vi "Forebrain - Bill.vi"() -> ()   [LabVIEW 2012]
doc: "This VI contrains the Forebrain within the Olin Robot Architecture. It must be run first to load the appropriate mission definition files. It contains a finite state machine built around a tabbed Operator interface that will guide an operator through the startup, run shutdown mission sequence. After running it, run the Midbrain and Hindbrain VIS."
panel:
  out "NXT String Sent":string="$B^"
  in  "Soft E-Stop":bool
  out "NXT String Received":string
  out "return count":u32
  out "error out":errorcluster
  in  "error in 2":errorcluster
  out "Desired \nVelocity":i16=5
  out "Local\nHeading":i16=90
  out "Ycurrent":dbl format="%#_3g"
  out "Xcurrent":dbl format="%#_3g"
  out "Ystart":dbl
  out "Xstart":dbl
  in  "error in":errorcluster
  out "Robot Live":bool
  in  "E-Stop":bool
  in  "Tab":T1(tab)
  out "MissionTime (Min)":dbl(knob) scale=0.0..10.0
  out "LidarDist":i16
  out "IR Index":i32
  out "BatteryLevel":dbl(slide) scale=6.0..9.0
  out "String Received":string
  out "Send String":string="$B^"
  in  "VISA resource name":refnum<visa-resource-name>="COM6"
  in  "Mode":i16 min=0 max=99 step=1
  in  "Desired Vel":i16(slide)=7 scale=0.0..14.0
  in  "Local Head":i16(slide)=7 scale=0.0..14.0
  out "StartMissionMap":picture
  out "MapDARCheck":picture
  in  "RunRobot":bool
  in  "Tug letter":string="G"
  out "Tug X":i32
  out "Tug Y":i32
  out "Tug H":i32
  out "BS Time Out?":bool
  out "Buoy locations":cluster{"regular expression":string, i32, i32}[](array[cluster])
  out "Valid ?":bool
  out "Battery\nVolts":i16
  out "Base Station data rec'd":string
  out "udp rate":bool
  out "CollisionWarning":bool
  out "DebugMapDAR":picture
  in  "MapDAR Control":T2={"NumberOfBeams"=180, "SensorRange"=500.0, "Noise (0.1 to 1)"=0.0} {"Noise (0.1 to 1)" min=0.0 max=1.0 step=0.1; "SensorRange" min=500.0 max=1500.0 step=100.0; "NumberOfBeams" min=36 max=360 step=2}
  out "MapDAR Data (r:pixel b:degrees)":cluster{"Range":dbl, "Bearing":dbl}[](array[cluster])
  in  "Stop DebugSENSE":bool
  out "MissionMap":picture
  out "Tug position":T3
  out "initialized MDF":T4(array[cluster])
  out "Way Point Index":i32
  out "InitialWaypoint":cluster{"X":i16, "Y":i16}
  in  "Pen Color":u32(colorbox)=15671808
  in  "Select Pen Attributes":T5={"Width"=1, "Style"=enum."Solid"}
  out "Draw??":bool
  in  "WhereAmI?FromBase":T6
  out "(xr,yr)":cluster{"X":dbl, "Y":dbl}
  in  "RobotPosition":T3 {"xrobot" min=0.0 max=1177.0 step=10.0; "yrobot" min=0.0 max=850.0 step=10.0; "heading" min=0.0 max=7.0 step=0.1}
  out "MDF_Original":T4(array[cluster])
  out "WhatAroundMeMap?":cluster{"T":dbl, "Range":dbl, "Bearing":dbl}[](array[cluster])
  out "WayPointAct":dbl[](array[numeric])
  out "SteerAngle":dbl
  out "MissionDefFile":picture
  out "MDF":T4(array[cluster])
  in  "Select Your Behavior":T7(ring)
  out "No. of Waypoints":i32
  in  "Exit Planning":bool
  in  "BoatSpeed for Leg":dbl(slide)=8.0 min=-9.0 max=9.0 step=1.0 scale=0.0..14.0
  out "BuildMDF":bool
  out "WayPoint Position":cluster{"X":i32, "Y":i32}
  in  "Upper Midbrain Active":bool
  out "Send String to NXT":string="$B^"
  in  "Behavior Command":T7(ring)
  out "CollisionLight":bool
  out "Where? Manual":T6
  out "ActManual":bool
  in  "Manual Heading":i16(knob) min=0 max=14 step=1
  out "MWhat?":bool
  out "Where? 2":bool
  out "How? 2":bool
  in  "ManualModeStop":bool
  out "ManualModeMapDAR":picture
  out "ManualMissionMap":picture
  out "Battery":dbl(slide) scale=0.0..8.0
  in  "Manual Vel":dbl(slide) min=0.0 max=14.0 step=1.0 scale=0.0..14.0
  out "MissionTime":dbl(knob) scale=0.0..10.0
  out "Heading":cluster{dbl, dbl}(knob)={0.0, 34.390870865624734} scale=180.0..-179.0 scale format="%#_3g"
  out "Speed":i16(knob) scale=-6.0..6.0
  out "Current Behavior":T7(ring)
  out "Robot Position":cluster{"X":dbl, "Y":dbl} {"X" format="%#_3g"; "Y" format="%#_3g"}
  out "Ready":bool
  in  "Pause":bool
  in  "Rerun MDF":bool
  out "CollisionLight 2":bool
  out "Act":bool
  out "Neo-C":bool
  out "How?":bool
  out "What?":bool
  out "A Heading":cluster{dbl, dbl}(knob)={0.0, 34.390870865624734} scale=180.0..-180.0
  out "A Speed":dbl(knob) scale=-9.0..9.0
  out "AutoBattery":dbl(slide) scale=0.0..8.0
  out "AutoModeLIDAR":picture
  out "AutoMissionMap":picture
  in  "RunAutoMode":bool
  out "MissionTimeAuto":dbl(knob) scale=0.0..60.0
  out "Where?":bool
  in  "Manual Override":bool
  in  "Destinations Array":i64[][](array[numeric])
  out "BAM Mission Map":picture
  in  "Pixel Y Goal":dbl
  in  "Pixel X Goal":dbl
  out "Pixel X":dbl
  out "Pixel Y":dbl
  out "Direction":dbl
  out "Base Station String":string
  out "Battery Level":dbl
  in  "Heading":i16(knob)=7
  in  "Velocity":i16(slide)=7 scale=0.0..14.0
  # "To run\nrobot,\nclick\narrow\nabove\n\nRun Robot button must be on"
  # "Operation Directions\n\n1)Click on Startup&\nShutdown tab.\n2) Click on Run \nArrow on menubar.\nRun Forebrain,\nvis from the project\nexplorer.\n3) Select a mssion \nmap file when asked.\n4) Check robot is \nfully operational on\nStartup tab.\n5) Debug with debug\ntabs as required.\n6) Select ManualMode\ntab and test drive \nrobot.\n7) Select PlanMission\ntab and set up \nmission.\n8) Go to AutoMode\ntab and run mission."
  # "Turns off drive\nmotors"
  # "Enter Olin Test  Pool"
  # "Xbee Com Port"
  # "xBee\"Send String\" (mode, desired velocity, local heading)"
  # "(Type in Tug Letter  L T G P  (look at boat cradle)"
  # "Should be on to\nrun"
  # "BoatG,X,Y,H,BoatT,X,Y,H,BoatP,X,Y.H,BoatL,X,Y,H,BuoyA,X,Y,BuoyB,X,Y,BuoyC,X,Y,BuoyD,X,Y,Time(hours,Min,Sec)"
  # "To stop  program \nturn off here"
  # "Use this tab\nto explore\nLIDAR\ndata and \noperation"
  # "Set\nNumberOfBeams\nSensorRange\nNoise\nto\nview\nsimulated\nsensor\ndata"
  # "Turn Debug Sim \nto leave this\ntab--->"
  # "This tab will auto\nreturn to Startup \nin 2 seconds"
  # "Clean up interface and make more useful for debugging behaviors"
  # "Build out interface and make more useful for debugging act"
  # "This tab will auto\nreturn to Startup \nin 2 seconds"
  # "Directions:\n1) Select Robot Behavior for each mission leg.\n2) Select Robot Speed for leg.\n3) Click on robots current location for first waypoint.\n4) Hold down button and drag to next\nwaypoint. Click on next leg waypoint.\n5) Hold mouse button down and drag to \nnext waypoint. \n6) Click on next waypoint. Repeat for full mission.\n7) MDF will store up to 20 waypoints."
  # "Remember to\nset boat\nleg speed !"
  # "Please Adjust Scroll Barrs in Tug Off Mode to Prevent  Extra Lines Being Drawn"
  # "\"Send String\" (mode, desired velocity, local heading)"
  # "Press to stop and return to StartUp"
  # "Open MidBrain\nArbiter to see\nBrain Waves"
  # "AutoMode\nAutomatically \nReturns to \nStartUp Mode"
  # "Pixel coordinates for destinations."
  # "BoatG,X,Y,H,BoatT,X,Y,H,BoatP,X,Y.H,BoatL,X,Y,H,BuoyA,X,Y,BuoyB,X,Y,BuoyC,X,Y,BuoyD,X,Y,Time(hours,Min,Sec)"
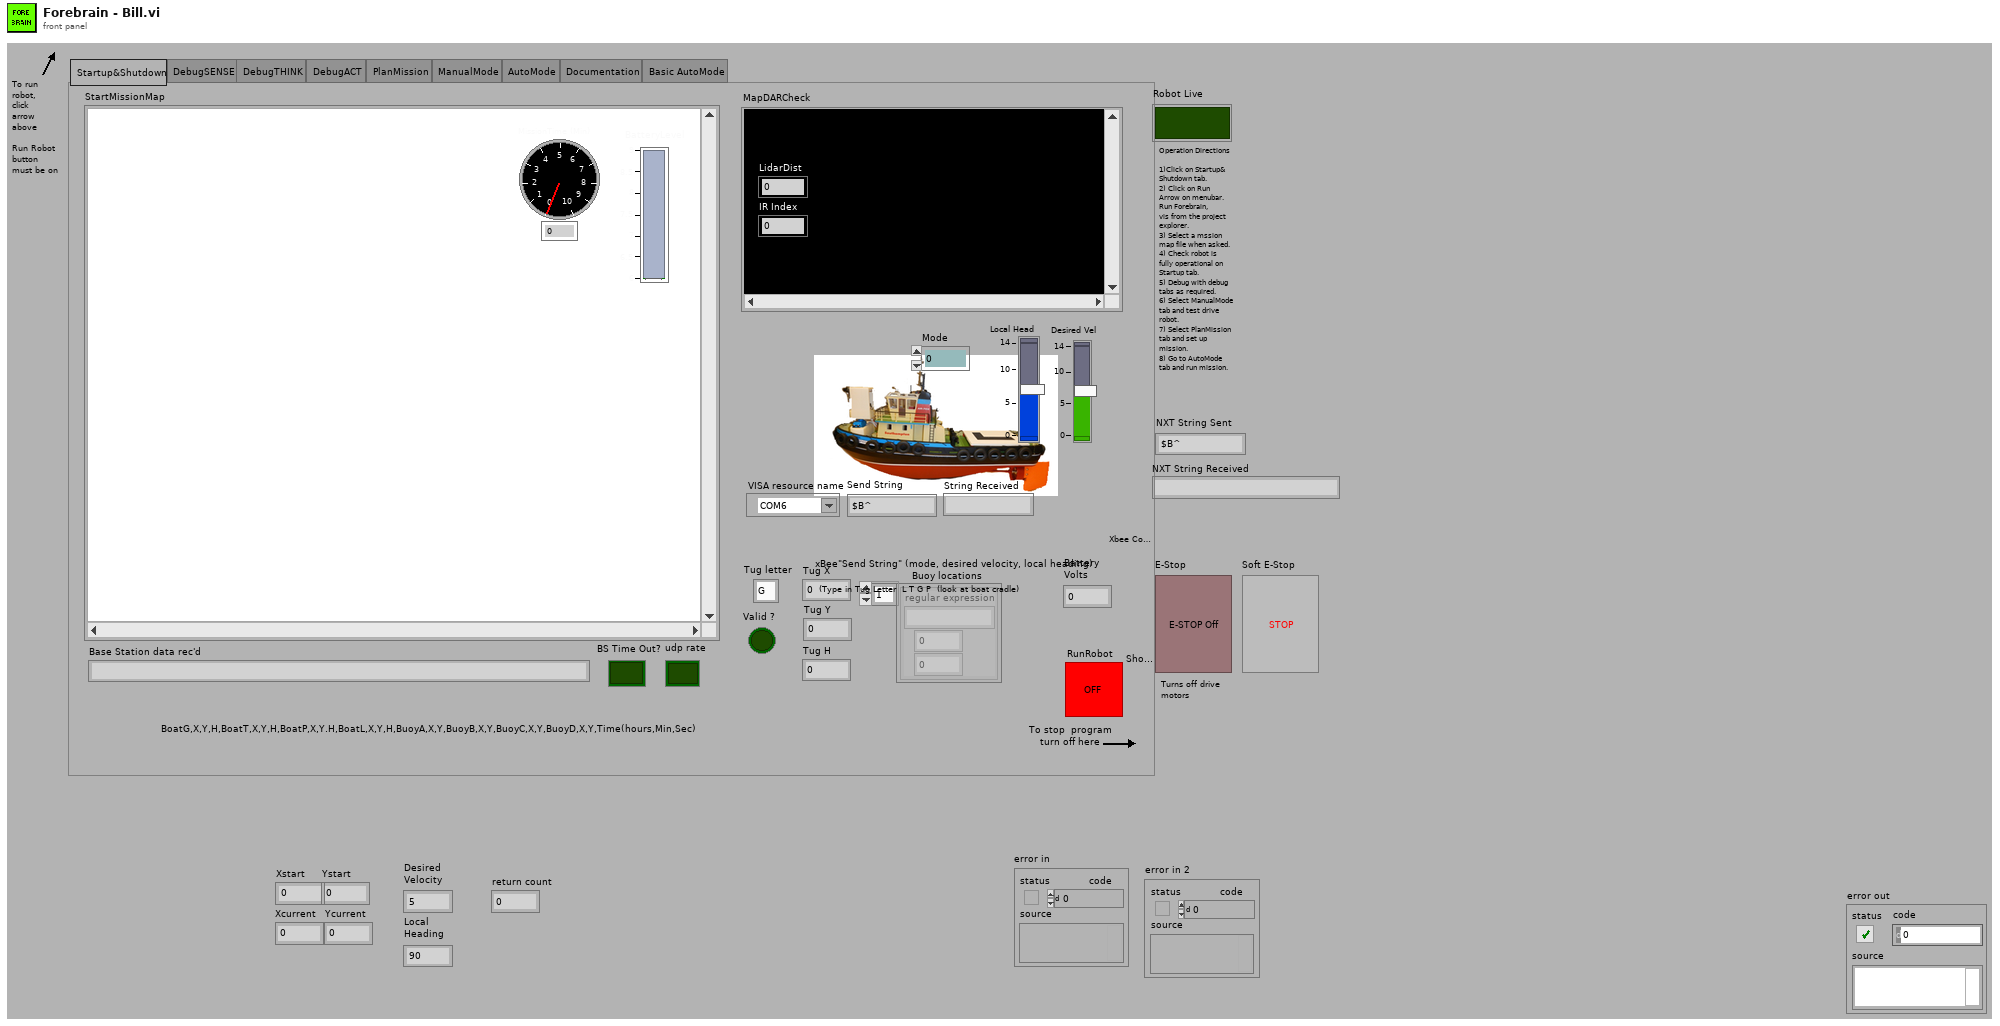
[diagram p1: front panel]
types:
  T1 = enum32{"Startup&Shutdown", "DebugSENSE", "DebugTHINK", "DebugACT", "PlanMission", "ManualMode", "AutoMode", "Documentation", "Basic AutoMode"}
  T2 = cluster{"NumberOfBeams":i32, "SensorRange":dbl, "Noise (0.1 to 1)":dbl}
  T3 = cluster{"xrobot":dbl, "yrobot":dbl, "heading":dbl}
  T4 = cluster{"Status":enum16{"Past", "Current", "Future"}, "x":dbl, "y":dbl, "z":dbl, "Vel":dbl, "Dwell Time":dbl, "BehCom":enum16{"Tug Off", "Manual Mode", "Goto WayPoint", "Back Up", "Circle", "Left Wall Follow", "Right Wall Follow", "Hunt"}, "Expand1":dbl, "Expand2":dbl, "Expand3":dbl}[]
  T5 = cluster{"Width":u16, "Style":enum32{"Solid", "Dash", "Dot", "DashDot", "DashDotDot"}}
  T6 = cluster{"T":dbl, "X":dbl, "Y":dbl, "Direction":dbl}
  T7 = enum16{"Tug Off", "Manual Mode", "Goto WayPoint", "Back Up", "Circle", "Left Wall Follow", "Right Wall Follow", "Hunt"}
  T8 = enum32{"Startup&Shutdown", "DebugSENSE", "DebugTHINK", "DebugACT", "PlanMission", "ManualMode", "AutoMode", "Documentation"}
  T9 = cluster{"VelCom":dbl, "BehCom":enum16{"OpenFieldTransit", "P-WallFollow", "S-WallFollow", "LaneFollow", "ManualMode"}}
  T10 = typedef "IMAQ Image.ctl" = refnum<image>
  T11 = typedef "imagedata.ctl" = cluster{"image type":i32, "image depth":i32, "image":u8[], "mask":u8[], "colors":u32[], "Rectangle":cluster{"left":i16, "top":i16, "right":i16, "bottom":i16}}
  T12 = cluster{"Status":enum16{"Past", "Current", "Future"}, "x":dbl, "y":dbl, "z":dbl, "Vel":dbl, "Dwell Time":dbl, "BehCom":enum16{"Tug Off", "Manual Mode", "Goto WayPoint", "Back Up", "Circle", "Left Wall Follow", "Right Wall Follow", "Hunt"}, "Expand1":dbl, "Expand2":dbl, "Expand3":dbl}
  T13 = typedef "LVMouseTypeDef.ctl" = cluster{"Mouse Position":cluster{"X":i32, "Y":i32}, "Mouse Modifiers":cluster{"Button Down":bool, "Shift Mod":bool, "Menu Mod":bool, "Option Mod":bool}}
  T14 = cluster{"regular expression":string, i32, i32, i32}
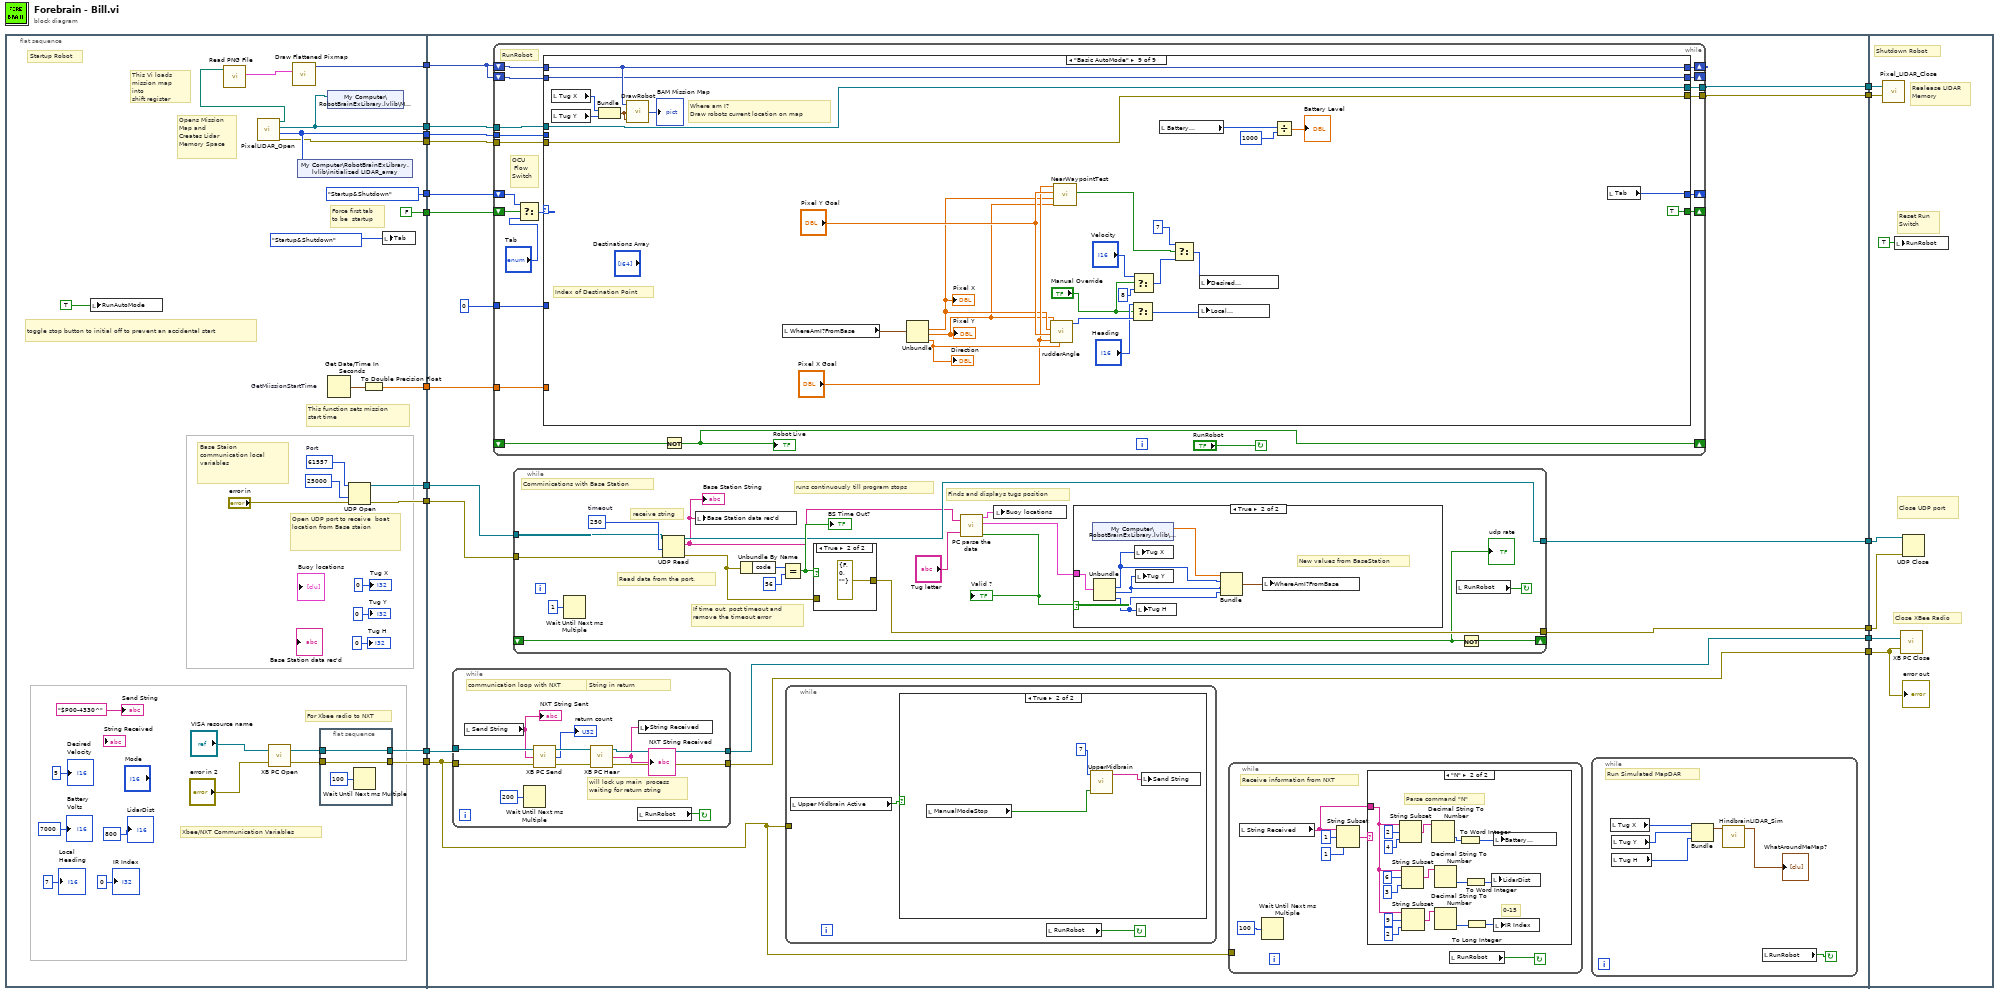
[diagram p0: block diagram]
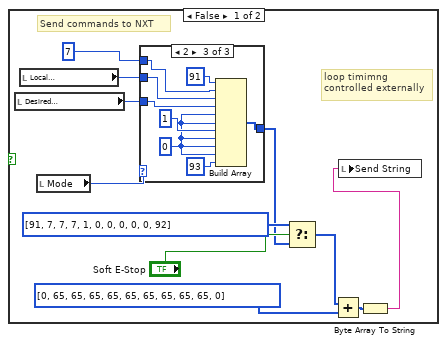
[diagram p3: hidden frame]
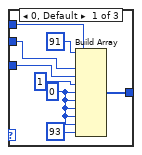
[diagram p4: hidden frame]
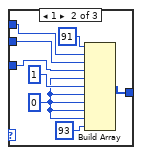
[diagram p5: hidden frame]
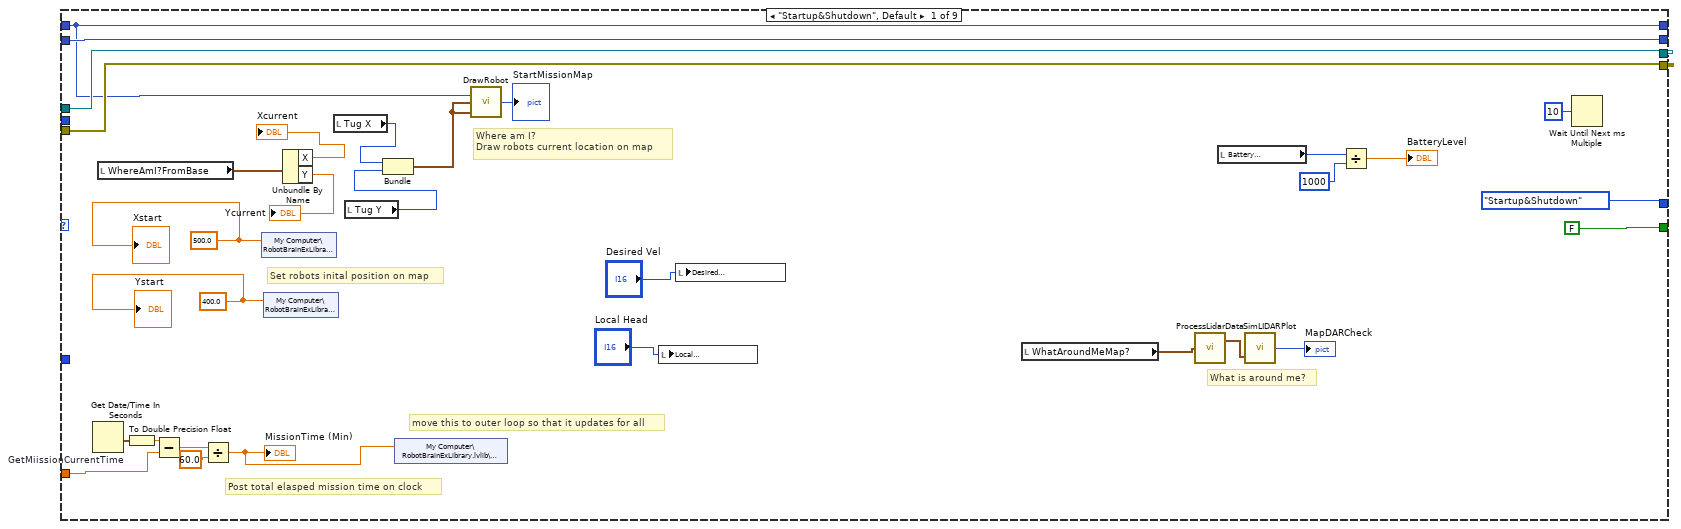
[diagram p8: hidden frame]
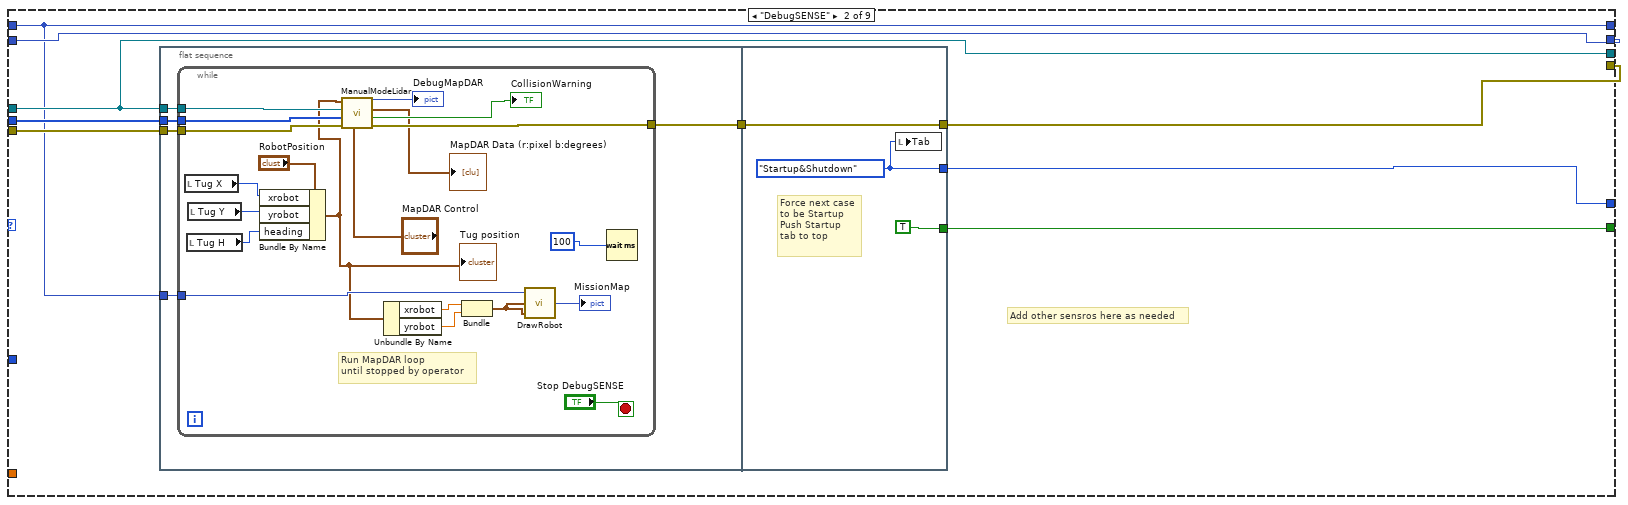
[diagram p9: hidden frame]
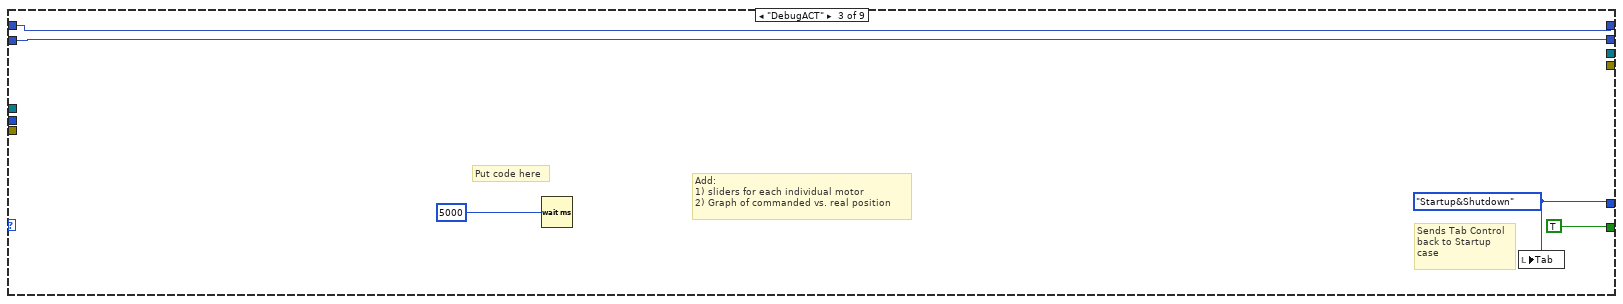
[diagram p10: hidden frame]
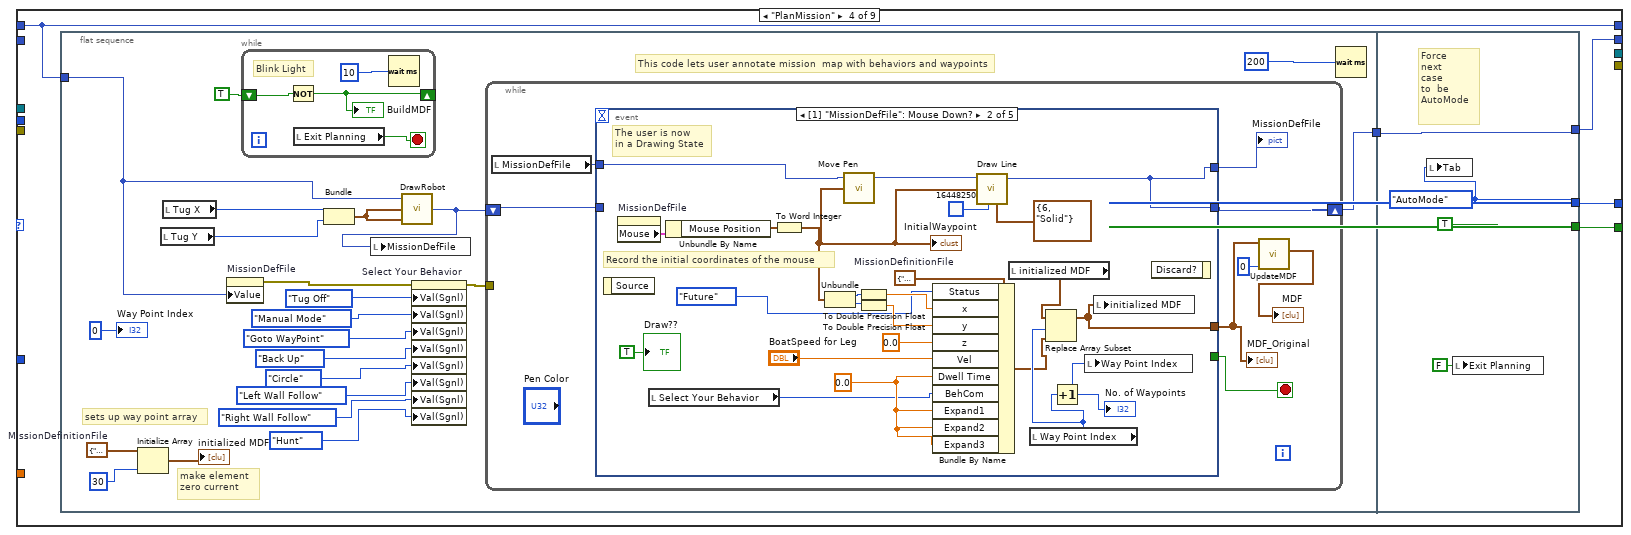
[diagram p11: hidden frame]
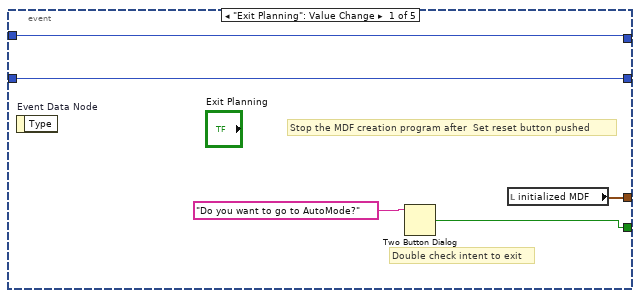
[diagram p12: hidden frame]
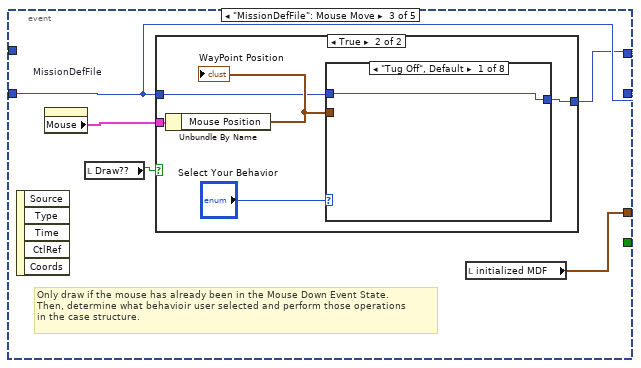
[diagram p13: hidden frame]
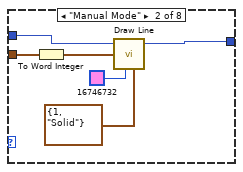
[diagram p15: hidden frame]
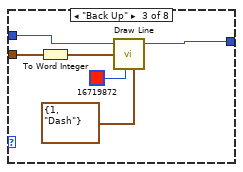
[diagram p16: hidden frame]
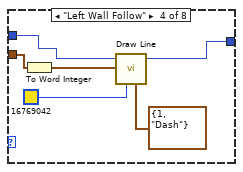
[diagram p17: hidden frame]
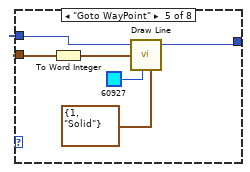
[diagram p18: hidden frame]
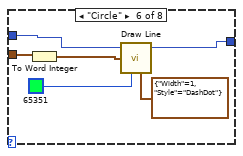
[diagram p19: hidden frame]
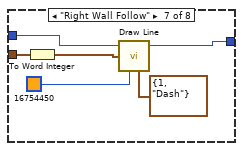
[diagram p20: hidden frame]
diagram:
  n1 = flat-sequence {
    tunnel: [w48] -> w17
    tunnel: [w47] -> w16
    tunnel: [w44] -> w15
    tunnel: [w46] -> w14
    tunnel: [w45] -> w13
    tunnel: [FALSE ("RunAutoMode")] -> w10
    tunnel: [T8."Startup&Shutdown" ("Tab")] -> w9
    tunnel: [w31] -> w8
    tunnel: [w30] -> w7
    tunnel: [w19] -> w6
    tunnel: [w18] -> w5
    tunnel: w17 -> [w70]
    tunnel: w16 -> [w69]
    tunnel: w15 -> [w68]
    tunnel: w14 -> [w67]
    tunnel: w13 -> [w66]
    tunnel: [w65] -> w12
    tunnel: [w64] -> w11
    tunnel: w10 -> [w63]
    tunnel: w9 -> [w62]
    tunnel: w8 -> [w57]
    tunnel: w7 -> [w56]
    tunnel: w6 -> [w61]
    tunnel: w5 -> [w58]
    tunnel: [w60] -> w4
    tunnel: [w59] -> w3
    tunnel: [w55] -> w2
    tunnel: [w54] -> w1
    tunnel: w12 -> [w647]
    tunnel: w11 -> [w646]
    tunnel: w4 -> [w645]
    tunnel: w3 -> [w644]
    tunnel: w2 -> [w643]
    tunnel: w1 -> [w642]
    frame #0 {
      w37 = u16 61557  # Port
      # "For Xbee radio to NXT"
      # "Xbee/NXT Communication Variables"
      # "Base Staion communication local variables"
      # "Open UDP port to receive  boat location from Base staion"
      # "Force first tab\nto be  startup"
      # "toggle stop button to initial off to prevent an accidental start"
      # "Opens Mission\nMap and\nCreates Lidar\nMemory Space"
      # "This function sets mission \nstart time"
      # "This Vi loads\nmission map into \nshift register"
      # "Startup Robot"
      n2 = local write "RunAutoMode"(TRUE ("RunAutoMode")) -> ()
      n3 = call "PixelLIDAR_Open.vi"() -> ("error out"=w45:errorcluster, "initialized LIDAR\narray"=w46:i32[], "MDF Image"=w44:T10, "MissionMap"=w39:path)  [unwired: 2 in]
      n4 = call <vilib>:"Read PNG File.vi"("path to PNG file"=w39) -> ("image data"=w38:T11)  [unwired: 8 in, 2 out]
      n5 = call "XB PC Open.vi"("error in (no error)"="error in 2", "VISA resource name"="VISA resource name") -> ("error out"=w22:errorcluster, "VISA resource name out"=w23:refnum<visa-resource-name>)
      n6 = call <vilib>:"Draw Flattened Pixmap.vi"("image data"=w38) -> ("new picture"=w47:picture)  [unwired: 8 in]
      n7 = shared-variable "My Computer\\RobotBrainExLibrary.lvlib\\initialized LIDAR_array"(w46) -> ()  [unwired: 1 in, 1 out]
      n8 = flat-sequence {
        tunnel: w23 -> [w50]
        tunnel: w22 -> [w51]
        tunnel: [w51] -> w18
        tunnel: [w50] -> w19
        frame #0 {
          n9 = Wait Until Next ms Multiple(millisecond multiple=u32 100) -> ()  [unwired: 1 out]
        }
      }
      n10 = shared-variable "My Computer\\RobotBrainExLibrary.lvlib\\MDF Image"(w44) -> ()  [unwired: 1 in, 1 out]
      n11 = Get Date/Time In Seconds "GetMiissionStartTime"() -> (seconds since 1Jan1904=w49:timestamp)
      n12 = UDP Open(8:"error in", 9:25000 ("timeout ms (25000)"), 11:w37) -> (port=w31:refnum<k16>, 0:w30:errorcluster)  [unwired: 2 in, 1 out]
      n13 = To Double Precision Float(number=w49) -> (double precision float=w48:dbl)
      n14 = local write "Tab"(T8."Startup&Shutdown" ("Tab")) -> ()
      "Tug X" <- 0 ("Tug X")
      "Tug Y" <- 0 ("Tug Y")
      "Tug H" <- 0 ("Tug H")
      "Battery\nVolts" <- i16 7000 ("Battery\nVolts")
      "LidarDist" <- i16 800 ("Dist")
      "IR Index" <- 0 ("IR Index")
      "Local\nHeading" <- i16 7 ("Local\nHeading")
      "Desired \nVelocity" <- i16 5 ("Desired \nVelocity")
      "Send String" <- "$P00-4330^"
    }
    frame #1 {
      n15 = while {
        tunnel: w61 -> [w149]
        tunnel: w58 -> [w148]
        tunnel: [w145] -> w59
        tunnel: [w144] -> w60
        stop <- w143 continue-if-true
        # "will lock up main  process\nwaiting for return string"
        # "communication loop with NXT"
        # "send a string to the NXT and receive a String in return"
        n16 = local read "Send String"() -> (w141:string)
        "NXT String Sent" <- w141
        n17 = Wait Until Next ms Multiple(millisecond multiple=u32 200) -> ()  [unwired: 1 out]
        n18 = call "XB PC Send.vi"("error in (no error)"=w148, "String"=w141, "VISA resource name"=w149) -> ("error out"=w147:errorcluster, "return count"=→"return count":u32, "VISA resource name out"=w146:refnum<visa-resource-name>)
        n19 = call "XB PC Hear.vi"("VISA resource name"=w146, "error in (no error)"=w147) -> ("VISA resource name out"=w144:refnum<visa-resource-name>, "String Received"=w140:string, "error out"=w145:errorcluster)
        "NXT String Received" <- w140
        n20 = local read "RunRobot"() -> (w143:bool)
        n21 = local write "String Received"(w140) -> ()
      }
      n22 = while {
        shift-right: [w178] -> _
        shift-left: _ -> [w194]
        shift-right: [w193] -> _
        shift-left: w62 -> [w192]
        shift-right: [w189] -> _
        shift-left: w63 -> [w188]
        tunnel: w70 -> [w187]
        shift-right: [w177] -> _
        shift-left: w69 -> [w186]
        shift-right: [w184] -> _
        shift-left: w69 -> [w185]
        tunnel: w68 -> [w183]
        tunnel: w67 -> [w182]
        tunnel: w66 -> [w181]
        tunnel: [w180] -> w65
        tunnel: [w179] -> w64
        tunnel: 0 -> [w176]
        stop <- "RunRobot" continue-if-true
        # "RunRobot"
        # "OCU\n Flow\nSwitch"
        n23 = Select(t=w192, s=w188, f="Tab") -> (s? t:f=w190:T1)
        n24 = case shown="\"Basic AutoMode\"" w190 {
          selector: w190 -> [_ _ _ _ _ w514 _ _ _]
          tunnel: [T8."Startup&Shutdown" ("Tab") w230 w265 w272 w439 w515 T8."Startup&Shutdown" ("Tab") w611 w629] -> w193
          tunnel: [FALSE ("s") w229 TRUE ("s") w271 w440 w513 FALSE ("s") TRUE ("s") TRUE ("s")] -> w189
          tunnel: w187 -> [w219 _ _ _ w437 w511 _ _ _]
          tunnel: w186 -> [w196 w226 w264 w268 w435 w508 w604 w609 w635]
          tunnel: w185 -> [w218 w227 w263 _ w436 w510 w603 w608 w634]
          tunnel: [w218 w227 w263 w269 w436 w510 w603 w608 w634] -> w184
          tunnel: w183 -> [w217 w228 _ _ _ _ _ _ w630]
          tunnel: w182 -> [_ w234 _ _ _ _ _ _ _]
          tunnel: w181 -> [w216 w233 _ _ _ _ _ _ w627]
          tunnel: [w217 w228 _ _ _ _ _ _ w630] -> w180
          tunnel: [w216 w232 _ _ _ _ _ _ w627] -> w179
          tunnel: [w196 w226 w264 w268 w435 w508 w604 w609 w635] -> w177
          tunnel: w176 -> [_ _ _ _ _ _ _ _ _]
          frame "Startup&Shutdown", Default {
            w208 = 400.0 ("Ystart")
            w209 = 500.0 ("Xstart")
            # "move this to outer loop so that it updates for all"
            # "Where am I?\nDraw robots current location on map"
            # "Post total elasped mission time on clock"
            # "What is around me?"
            # "Set robots inital position on map"
            n25 = Get Date/Time In Seconds "GetMiissionCurrentTime"() -> (seconds since 1Jan1904=w223:timestamp)
            n26 = local read "WhereAmI?FromBase"() -> (w197:T6)
            n27 = To Double Precision Float(number=w223) -> (double precision float=w222:dbl)
            n28 = Subtract(x=w222, y=w219) -> (x-y=w221:dbl)
            n29 = Divide(x=w221, y=60.0) -> (x/y=w215:dbl)
            "MissionTime (Min)" <- w215
            n30 = shared-variable "My Computer\\RobotBrainExLibrary.lvlib\\Xstart"(w209) -> ()  [unwired: 1 in, 1 out]
            n31 = shared-variable "My Computer\\RobotBrainExLibrary.lvlib\\Ystart"(w208) -> ()  [unwired: 1 in, 1 out]
            n32 = Unbundle By Name(w197) -> ("X"=→"Xcurrent":dbl, "Y"=→"Ycurrent":dbl)
            n33 = local read "Tug X"() -> (w207:i32)
            n34 = local read "Tug Y"() -> (w206:i32)
            n35 = Bundle("Tug X"=w207, "Tug Y"=w206) -> (w212:cluster{"Tug X":i32, "Tug Y":i32})  [unwired: 1 in]
            n36 = shared-variable "My Computer\\RobotBrainExLibrary.lvlib\\MissionTime"(w215) -> ()  [unwired: 1 in, 1 out]
            n37 = call "DrawRobot.vi"("(xr,yr) old"=w212, "(xr,yr) new"=w212, "2D Picture"=w196) -> ("new picture"=→"StartMissionMap":picture)
            n38 = local write "Local\nHeading"("Local Head") -> ()
            n39 = local write "Desired \nVelocity"("Desired Vel") -> ()
            n40 = local read "WhatAroundMeMap?"() -> (w198:cluster{"T":dbl, "Range":dbl, "Bearing":dbl}[])
            n41 = call "ProcessLidarData.vi"("WhatAroundMe?MM"=w198) -> ("data array [mag, phase (deg)]"=w213:cluster{"magnitude":dbl, "phase":dbl}[])  [unwired: 1 out]
            n42 = local read "Battery\nVolts"() -> (w203:i16)
            n43 = call "SimLIDARPlot.vi"("data array [mag, phase (deg)]"=w213) -> ("SONAR"=→"MapDARCheck":picture)  [unwired: 1 in]
            n44 = Divide(x=w203, y=i16 1000) -> (x/y=→"BatteryLevel":dbl)
            n45 = Wait Until Next ms Multiple(millisecond multiple=u32 10) -> ()  [unwired: 1 out]
            "Xstart" <- w209
            "Ystart" <- w208
          }
          frame "DebugSENSE" {
            # "Add other sensros here as needed"
            n46 = flat-sequence {
              tunnel: w234 -> [w239]
              tunnel: w233 -> [w238]
              tunnel: w228 -> [w237]
              tunnel: [w236] -> w231
              tunnel: w226 -> [w235]
              tunnel: [w262] -> w232
              tunnel: w231 -> [w262]
              tunnel: [w261] -> w230
              tunnel: [TRUE ("s")] -> w229
              frame #0 {
                n47 = while {
                  tunnel: w239 -> [w259]
                  tunnel: w238 -> [w258]
                  tunnel: w237 -> [w257]
                  tunnel: [w256] -> w236
                  tunnel: w235 -> [w250]
                  stop <- "Stop DebugSENSE" stop-if-true
                  # "Run MapDAR loop\nuntil stopped by operator"
                  n48 = local read "Tug X"() -> (w244:i32)
                  n49 = local read "Tug H"() -> (w245:i32)
                  n50 = local read "Tug Y"() -> (w243:i32)
                  n51 = Bundle By Name(cluster="RobotPosition", "xrobot"=w244, "yrobot"=w243, "heading"=w245) -> (w241:T3)
                  "Tug position" <- w241
                  n52 = call "ManualModeLidar.vi"("LIDARControl"="MapDAR Control", "error in"=w258, "initialized \nsonar ray\narray"=w259, "MDF Image"=w257, "SubPosition"=w241) -> ("error out"=w256:errorcluster, "Collision\nWarning"=→"CollisionWarning":bool, "LIDAR Data (r:pixel b:degrees)"=→"MapDAR Data (r:pixel b:degrees)":cluster{"Range":dbl, "Bearing":dbl}[], "LIDAR"=→"DebugMapDAR":picture)  [unwired: 1 in]
                  n53 = Unbundle By Name(w241) -> ("xrobot"=w248:dbl, "yrobot"=w247:dbl)
                  n54 = Bundle("xrobot"=w248, "yrobot"=w247) -> (w240:cluster{"xrobot":dbl, "yrobot":dbl})  [unwired: 1 in]
                  n55 = call "DrawRobot.vi"("(xr,yr) old"=w240, "(xr,yr) new"=w240, "2D Picture"=w250) -> ("new picture"=→"MissionMap":picture)
                  n56 = Wait (ms)(milliseconds to wait=u32 100) -> ()  [unwired: 1 out]
                }
              }
              frame #1 {
                w261 = T8."Startup&Shutdown" ("Tab")
                # "Force next case\nto be Startup\nPush Startup\ntab to top"
                n57 = local write "Tab"(w261) -> ()
              }
            }
          }
          frame "DebugACT" {
            w265 = T8."Startup&Shutdown" ("Tab")
            # "Add:\n1) sliders for each individual motor\n2) Graph of commanded vs. real position"
            # "Put code here"
            # "Sends Tab Control\nback to Startup\ncase"
            n58 = Wait (ms)(milliseconds to wait=u32 5000) -> ()  [unwired: 1 out]
            n59 = local write "Tab"(w265) -> ()
          }
          frame "PlanMission" {
            n60 = flat-sequence {
              tunnel: [w293] -> w270
              tunnel: w268 -> [w286]
              tunnel: [w433] -> w272
              tunnel: [TRUE ("s")] -> w271
              tunnel: w270 -> [w432]
              tunnel: [w432] -> w269
              frame #0 {
                w284 = T12 {"Status"=enum."Future", "x"=0.0, "y"=0.0, "z"=0.0, "Vel"=0.0, "Dwell Time"=0.0, "BehCom"=enum."Tug Off", "Expand1"=0.0, "Expand2"=0.0, "Expand3"=0.0}  # MissionDefinitionFile
                # "make element \nzero current"
                # "sets up way point array"
                # "This code lets user annotate mission  map with behaviors and waypoints"
                n61 = Initialize Array ("Initialize WaypointArray")(w284, 30 ("dimension size")) -> (→"initialized MDF":T4)
                n62 = local read "Tug Y"() -> (w281:i32)
                n63 = local read "Tug X"() -> (w282:i32)
                n64 = property on="MissionDefFile" class="Pict"("Value"=w286) -> (error out=w291:errorcluster)  [unwired: 2 in, 1 out]
                n65 = while {
                  shift-right: [w297] -> _
                  shift-left: TRUE -> [w298]
                  stop <- w296 stop-if-true
                  # "Blink Light"
                  n66 = Not(x=w298) -> (.not. x?=w297:bool)
                  "BuildMDF" <- w297
                  n67 = local read "Exit Planning"() -> (w296:bool)
                  n68 = Wait (ms)(milliseconds to wait=u32 10) -> ()  [unwired: 1 out]
                }
                n69 = Bundle("Tug X"=w282, "Tug Y"=w281) -> (w287:cluster{"Tug X":i32, "Tug Y":i32})  [unwired: 1 in]
                n70 = call "DrawRobot.vi"("(xr,yr) old"=w287, "(xr,yr) new"=w287, "2D Picture"=w286) -> ("new picture"=w285:picture)
                n71 = local write "MissionDefFile"(w285) -> ()
                n72 = property on="Select Your Behavior" class="Enum (strict)"(error in=w291, "Val(Sgnl)"=T7."Tug Off" ("Value (Signaling)"), "Val(Sgnl)"=T7."Manual Mode" ("Value (Signaling)"), "Val(Sgnl)"=T7."Goto WayPoint" ("Value (Signaling)"), "Val(Sgnl)"=T7."Back Up" ("Value (Signaling)"), "Val(Sgnl)"=T7."Circle" ("Value (Signaling)"), "Val(Sgnl)"=T7."Left Wall Follow" ("Value (Signaling)"), "Val(Sgnl)"=T7."Right Wall Follow" ("Value (Signaling)"), "Val(Sgnl)"=T7."Hunt" ("Value (Signaling)")) -> (error out=w292:errorcluster)  [unwired: 1 in, 1 out]
                n73 = while {
                  shift-right: [w305] -> w293
                  shift-left: w285 -> [w306]
                  tunnel: w292 -> [_]
                  stop <- w304 stop-if-true
                  n74 = local read "MissionDefFile"() -> (w303:picture)
                  n75 = event shown="[1] \"MissionDefFile\": Mouse Down?" {
                    selector: _ -> [_ _ _ _ _]
                    dyn-events: _ -> [_ _ _ _ _]
                    timeout: _ -> [_ _ _ _ _]
                    tunnel: [w309 w317 w337 w390 w428] -> w305
                    tunnel: w306 -> [w309 _ w337 w390 _]
                    tunnel: [w310 _ _ _ _] -> w304
                    tunnel: [w308 w332 w338 w392 w429] -> w300
                    tunnel: w303 -> [w307 w318 _ w391 w428]
                    tunnel: [w307 w317 w336 w391 w428] -> w302
                    event "Exit Planning": Value Change {
                      # "Double check intent to exit"
                      # "Stop the MDF creation program after  Set reset button pushed"
                      n76 = event-data "Event Data Node"() -> ()  [unwired: 1 in, 1 out]
                      n77 = Two Button Dialog(message="Do you want to go to AutoMode?") -> (T button?=w310:bool)  [unwired: 2 in]
                      n78 = local read "initialized MDF"() -> (w308:T4)
                    }
                    event "MissionDefFile": Mouse Down? {
                      w316 = T12 {"Status"=enum."Future", "x"=0.0, "y"=0.0, "z"=0.0, "Vel"=0.0, "Dwell Time"=0.0, "BehCom"=enum."Tug Off", "Expand1"=0.0, "Expand2"=0.0, "Expand3"=0.0}  # MissionDefinitionFile
                      w326 = 0.0 ("Dwell Time")
                      # "Record the initial coordinates of the mouse"
                      # "The user is now\nin a Drawing State"
                      n79 = event-data() -> ()  [unwired: 1 in, 1 out]
                      n80 = property on="MissionDefFile" class="Pict"() -> ("Mouse"=w335:T13)  [unwired: 2 in, 2 out]
                      n81 = local read "Select Your Behavior"() -> (w313:T7)
                      n82 = Unbundle By Name(w335) -> ("Mouse Position"=w333:cluster{"X":i32, "Y":i32})
                      n83 = To Word Integer(number=w333) -> (16bit integer=w321:cluster{"X":i16, "Y":i16})
                      "InitialWaypoint" <- w321
                      n84 = Unbundle(w321) -> ("X"=w330:i16, "Y"=w329:i16)
                      n85 = call <vilib>:"Move Pen.vi"("new position"=w321, "picture"=w318) -> ("new picture"=w322:picture)  [unwired: 3 in]
                      n86 = To Double Precision Float(number=w330) -> (double precision float=w328:dbl)
                      n87 = To Double Precision Float(number=w329) -> (double precision float=w327:dbl)
                      n88 = Bundle By Name(cluster=w316, "Status"=enum16{"Past", "Current", "Future"}."Future", "x"=w328, "y"=w327, "z"=0.0, "Vel"="BoatSpeed for Leg", "Dwell Time"=w326, "BehCom"=w313, "Expand1"=w326, "Expand2"=w326, "Expand3"=w326) -> (w312:T12)
                      n89 = call <vilib>:"Draw Line.vi"("picture"=w322, "end point"=w321, "color(black)"=u32 16448250, "pen"=T5 {"Width"=6, "Style"=enum."Solid"}) -> ("new picture"=w317:picture)  [unwired: 5 in]
                      n90 = local read "initialized MDF"() -> (w331:T4)
                      n91 = local read "Way Point Index"() -> (w314:i32)
                      n92 = Replace Array Subset(array=w331, new element=w312, index=w314) -> (w332:T4)
                      n93 = Increment(x=w314) -> (x+1=w334:i32)
                      "No. of Waypoints" <- w334
                      n94 = local write "Way Point Index"(w334) -> ()
                      n95 = local write "initialized MDF"(w332) -> ()
                      n96 = event-data() -> ()  [unwired: 2 in, 1 out]
                      "Draw??" <- TRUE ("Draw??")
                    }
                    event "MissionDefFile": Mouse Move {
                      # "Only draw if the mouse has already been in the Mouse Down Event State.\nThen, determine what behavioir user selected and perform those operations\nin the case structure."
                      n97 = event-data() -> ()  [unwired: 1 in, 5 out]
                      n98 = property on="MissionDefFile" class="Pict"() -> ("Mouse"=w340:T13)  [unwired: 2 in, 2 out]
                      n99 = local read "Draw??"() -> (w339:bool)
                      n100 = case shown="True" w339 {
                        tunnel: w340 -> [_ w346]
                        tunnel: w337 -> [w341 w342]
                        tunnel: [w341 w343] -> w336
                        frame False {
                        }
                        frame True {
                          n101 = Unbundle By Name(w346) -> ("Mouse Position"=w344:cluster{"X":i32, "Y":i32})
                          "WayPoint Position" <- w344
                          n102 = case shown="\"Tug Off\", Default" "Select Your Behavior" {
                            tunnel: w344 -> [_ w352 w358 w361 w367 w372 w378 w384]
                            tunnel: [w347 w353 w359 w363 w366 w373 w379 w385] -> w343
                            tunnel: w342 -> [w347 w351 w355 w364 w368 w374 w380 w386]
                            frame "Tug Off", Default {
                            }
                            frame "Manual Mode" {
                              n103 = To Word Integer(number=w352) -> (16bit integer=w348:cluster{"X":i16, "Y":i16})
                              n104 = call <vilib>:"Draw Line.vi"("picture"=w351, "end point"=w348, "color(black)"=u32 16746732, "pen"=T5 {"Width"=1, "Style"=enum."Solid"}) -> ("new picture"=w353:picture)  [unwired: 5 in]
                            }
                            frame "Back Up" {
                              n105 = To Word Integer(number=w358) -> (16bit integer=w354:cluster{"X":i16, "Y":i16})
                              n106 = call <vilib>:"Draw Line.vi"("picture"=w355, "end point"=w354, "color(black)"=u32 16719872, "pen"=T5 {"Width"=1, "Style"=enum."Dash"}) -> ("new picture"=w359:picture)  [unwired: 5 in]
                            }
                            frame "Left Wall Follow" {
                              n107 = To Word Integer(number=w361) -> (16bit integer=w362:cluster{"X":i16, "Y":i16})
                              n108 = call <vilib>:"Draw Line.vi"("picture"=w364, "end point"=w362, "color(black)"=u32 16769042, "pen"=T5 {"Width"=1, "Style"=enum."Dash"}) -> ("new picture"=w363:picture)  [unwired: 5 in]
                            }
                            frame "Goto WayPoint" {
                              n109 = To Word Integer(number=w367) -> (16bit integer=w369:cluster{"X":i16, "Y":i16})
                              n110 = call <vilib>:"Draw Line.vi"("picture"=w368, "end point"=w369, "color(black)"=u32 60927, "pen"=T5 {"Width"=1, "Style"=enum."Solid"}) -> ("new picture"=w366:picture)  [unwired: 5 in]
                            }
                            frame "Circle" {
                              n111 = To Word Integer(number=w372) -> (16bit integer=w377:cluster{"X":i16, "Y":i16})
                              n112 = call <vilib>:"Draw Line.vi"("picture"=w374, "end point"=w377, "color(black)"=u32 65351, "pen"=T5 {"Width"=1, "Style"=enum."DashDot"}) -> ("new picture"=w373:picture)  [unwired: 5 in]
                            }
                            frame "Right Wall Follow" {
                              n113 = To Word Integer(number=w378) -> (16bit integer=w383:cluster{"X":i16, "Y":i16})
                              n114 = call <vilib>:"Draw Line.vi"("picture"=w380, "end point"=w383, "color(black)"=u32 16754450, "pen"=T5 {"Width"=1, "Style"=enum."Dash"}) -> ("new picture"=w379:picture)  [unwired: 5 in]
                            }
                            frame "Hunt" {
                              n115 = To Word Integer(number=w384) -> (16bit integer=w387:cluster{"X":i16, "Y":i16})
                              n116 = call <vilib>:"Draw Line.vi"("picture"=w386, "end point"=w387, "color(black)"=u32 16720896, "pen"=T5 {"Width"=1, "Style"=enum."DashDotDot"}) -> ("new picture"=w385:picture)  [unwired: 5 in]
                            }
                          }
                        }
                      }
                      n117 = local read "initialized MDF"() -> (w338:T4)
                    }
                    event "Select Your Behavior": Value Change {
                      # "When the user selects a new operation, we disable certain controls that aren't relevant to\nthe operation that the user is performing."
                      n118 = event-data() -> ("NewVal"=w395:T7)  [unwired: 1 in]
                      n119 = property on="Select Pen Attributes" class="Clust (strict)"() -> ("Controls[]"=w394:refnum<vi>[])  [unwired: 2 in, 2 out]
                      n120 = case shown="\"Manual Mode\"" w395 {
                        tunnel: w394 -> [w399 w400 w404 w408 w412 w416 w420 w424]
                        tunnel: "Select Pen Attributes" -> [_ _ _ _ _ _ _ _]
                        frame "Manual Mode" {
                          # "All attributes are valid for this\noperation."
                          n121 = Index Array "Index Array"(array=w399, index=1) -> (element=w397:refnum<vi>)
                          n122 = property on="Property Node" class="Ctl"(reference=w397, "Disabled"=u8 0) -> ()  [unwired: 1 in, 2 out]
                        }
                        frame "Back Up" {
                          # "All attributes are valid for this\noperation."
                          n123 = Index Array(array=w400, index=1) -> (element=w402:refnum<vi>)
                          n124 = property class="Ctl"(reference=w402, "Disabled"=u8 0) -> ()  [unwired: 1 in, 2 out]
                        }
                        frame "Tug Off" {
                          # "All attributes are valid for this\noperation."
                          n125 = Index Array "Index Array"(array=w404, index=1) -> (element=w406:refnum<vi>)
                          n126 = property on="Property Node" class="Ctl"(reference=w406, "Disabled"=u8 0) -> ()  [unwired: 1 in, 2 out]
                        }
                        frame "Left Wall Follow" {
                          # "All attributes are valid for this\noperation."
                          n127 = Index Array "Index Array"(array=w408, index=1) -> (element=w410:refnum<vi>)
                          n128 = property on="Property Node" class="Ctl"(reference=w410, "Disabled"=u8 0) -> ()  [unwired: 1 in, 2 out]
                        }
                        frame "Goto WayPoint" {
                          # "All attributes are valid for this\noperation."
                          n129 = Index Array "Index Array"(array=w412, index=1) -> (element=w414:refnum<vi>)
                          n130 = property on="Property Node" class="Ctl"(reference=w414, "Disabled"=u8 0) -> ()  [unwired: 1 in, 2 out]
                        }
                        frame "Circle" {
                          # "All attributes are valid for this\noperation."
                          n131 = Index Array "Index Array"(array=w416, index=1) -> (element=w418:refnum<vi>)
                          n132 = property on="Property Node" class="Ctl"(reference=w418, "Disabled"=u8 0) -> ()  [unwired: 1 in, 2 out]
                        }
                        frame "Right Wall Follow" {
                          # "All attributes are valid for this\noperation."
                          n133 = Index Array "Index Array"(array=w420, index=1) -> (element=w422:refnum<vi>)
                          n134 = property on="Property Node" class="Ctl"(reference=w422, "Disabled"=u8 0) -> ()  [unwired: 1 in, 2 out]
                        }
                        frame "Hunt" {
                          # "All attributes are valid for this\noperation."
                          n135 = Index Array "Index Array"(array=w424, index=1) -> (element=w426:refnum<vi>)
                          n136 = property on="Property Node" class="Ctl"(reference=w426, "Disabled"=u8 0) -> ()  [unwired: 1 in, 2 out]
                        }
                      }
                      n137 = local read "initialized MDF"() -> (w392:T4)
                    }
                    event "MissionDefFile": Mouse Up {
                      # "When the user is finished drawing, we complete the operation."
                      # "Finished Drawing"
                      n138 = event-data() -> ()  [unwired: 1 in, 3 out]
                      n139 = local write "Draw??"(FALSE ("Draw??")) -> ()
                      n140 = local read "initialized MDF"() -> (w429:T4)
                    }
                  }
                  "MissionDefFile" <- w302
                  "MDF_Original" <- w300
                  n141 = call "UpdateMDF.vi"("Index"=0, "MDF_In"=w300) -> ("MDF_Out"=→"MDF":T4)  [unwired: 9 in]
                }
                n142 = Wait (ms)(milliseconds to wait=u32 200) -> ()  [unwired: 1 out]
                "Way Point Index" <- 0 ("Boundary Point Index")
              }
              frame #1 {
                w433 = T8."AutoMode" ("Tab")
                # "Force \nnext \ncase\nto  be\nAutoMode"
                n143 = local write "Tab"(w433) -> ()
                n144 = local write "Exit Planning"(FALSE ("Exit Planning")) -> ()
              }
            }
          }
          frame "ManualMode" {
            # "Removing map shift register\nfixed memory leak?"
            # "Manual Steering by dashboard heading steering wheel\nand by speed slider"
            # "This mode lets \noperator directly\ndrive robot via\nthe ManualMode\ntabbed interface"
            n145 = while {
              shift-right: [w463] -> _
              shift-left: _ -> [w462]
              tunnel: w437 -> [w455]
              shift-right: [w452] -> _
              shift-left: _ -> [w451]
              tunnel: w435 -> [w449]
              stop <- w461 stop-if-true
              # "WhereAmI?"
              n146 = Get Date/Time In Seconds "GetMiissionCurrentTime"() -> (seconds since 1Jan1904=w456:timestamp)
              n147 = call "WhereForebrainPerception.vi"("Where? Midbrain"="WhereAmI?FromBase") -> ("Where? Forebrain"=→"Where? Manual":T6, "(xr,yr)"=w452:cluster{"X":dbl, "Y":dbl}, "Direction"=w441:dbl)  [unwired: 3 in, 1 out]
              "(xr,yr)" <- w452
              n148 = local read "ManualModeStop"() -> (w461:bool)
              n149 = To Double Precision Float(number=w456) -> (double precision float=w457:dbl)
              n150 = Greater Or Equal?(x=w441, y=181.0) -> (x >= y?=w446:bool)
              n151 = local read "Manual Heading"() -> (w453:i16)
              n152 = Subtract(x=w457, y=w455) -> (x-y=w458:dbl)
              n153 = Not(x=w462) -> (.not. x?=w463:bool)
              n154 = call "DrawRobot.vi"("(xr,yr) old"=w451, "(xr,yr) new"=w452, "2D Picture"=w449) -> ("new picture"=→"ManualMissionMap":picture)
              n155 = Divide(x=w458, y=60.0) -> (x/y=w460:dbl)
              "MissionTime" <- w460
              n156 = Subtract(x=w441, y=360.0) -> (x-y=w444:dbl)
              n157 = shared-variable "My Computer\\RobotBrainExLibrary.lvlib\\MissionTime"(w460) -> ()  [unwired: 1 in, 1 out]
              n158 = Select(t=w444, s=w446, f=w441) -> (s? t:f=w443:dbl)
              n159 = Bundle("Direction"=w443, "Manual Heading"=w453) -> (→"Heading":cluster{"Direction":dbl, "Manual Heading":i16})  [unwired: 1 in]
              n160 = Wait Until Next ms Multiple(millisecond multiple=u32 100 ("milliseconds to wait")) -> ()  [unwired: 1 out]
              "Where? 2" <- w462
            }
            n161 = while {
              shift-right: [w470] -> _
              shift-left: _ -> [w471]
              stop <- "ManualModeStop" stop-if-true
              # "WhatIsAroundMe?"
              n162 = local read "WhatAroundMeMap?"() -> (w465:cluster{"T":dbl, "Range":dbl, "Bearing":dbl}[])
              n163 = call "ProcessLidarData.vi"("WhatAroundMe?MM"=w465) -> ("Collision"=w466:bool, "data array [mag, phase (deg)]"=w467:cluster{"magnitude":dbl, "phase":dbl}[])
              "CollisionLight" <- w466
              n164 = Not(x=w471) -> (.not. x?=w470:bool)
              "MWhat?" <- w470
              n165 = call "SimLIDARPlot.vi"("data array [mag, phase (deg)]"=w467) -> ("SONAR"=→"ManualModeMapDAR":picture)  [unwired: 1 in]
              n166 = case shown="True" w466 {
                frame False {
                  # "No \nBeep"
                }
                frame True {
                  n167 = call <vilib>:"Beep.vi"("use system alert? (T)"=TRUE, "duration (msec)"=u32 1000, "frequency (Hz)"=u32 900) -> ()  [unwired: 9 in]
                }
              }
              n168 = Wait Until Next ms Multiple(millisecond multiple=u32 100 ("milliseconds to wait")) -> ()  [unwired: 1 out]
            }
            n169 = while {
              shift-right: [w495] -> _
              shift-left: _ -> [w494]
              stop <- w493 stop-if-true
              # "HowAmI?"
              n170 = local read "Battery\nVolts"() -> (w492:i16)
              n171 = local read "ManualModeStop"() -> (w493:bool)
              n172 = Not(x=w494) -> (.not. x?=w495:bool)
              n173 = Divide(x=w492, y=i16 1000) -> (x/y=→"Battery":dbl)
              n174 = Wait Until Next ms Multiple(millisecond multiple=u32 100 ("milliseconds to wait")) -> ()  [unwired: 1 out]
              "How? 2" <- w494
            }
            n175 = while {
              shift-right: [w489] -> _
              shift-left: _ -> [w488]
              stop <- w487 stop-if-true
              # "ForebrainAct"
              n176 = local read "E-Stop"() -> (w485:bool)
              n177 = local read "ManualModeStop"() -> (w487:bool)
              n178 = Select(t=0.0, s=w485, f="Manual Vel") -> (s? t:f=w482:dbl)
              n179 = To Word Integer(number=w482) -> (16bit integer=w480:i16)
              "Speed" <- w480
              n180 = local read "Send String"() -> (→"Send String to NXT":string)
              n181 = To Word Integer(number="Behavior Command") -> (16bit integer=w477:i16)
              n182 = local write "Upper Midbrain Active"("Upper Midbrain Active") -> ()
              n183 = local write "Mode"(w477) -> ()
              n184 = local write "Desired \nVelocity"(w480) -> ()
              n185 = local write "Local\nHeading"("Manual Heading") -> ()
              n186 = Not(x=w488) -> (.not. x?=w489:bool)
              n187 = Wait Until Next ms Multiple(millisecond multiple=u32 50 ("milliseconds to wait")) -> ()  [unwired: 1 out]
              "ActManual" <- w488
            }
            n188 = local read "ManualModeStop"() -> (w438:bool)
            n189 = case shown="True" w438 {
              tunnel: [TRUE ("s") w499] -> w440
              tunnel: [T8."ManualMode" ("Tab") w500] -> w439
              frame False {
              }
              frame True {
                # "Debounce tab for clean transition"
                n190 = flat-sequence {
                  tunnel: [w506] -> w500
                  tunnel: [TRUE ("s")] -> w499
                  frame #0 {
                    n191 = Wait (ms)(milliseconds to wait=u32 100) -> ()  [unwired: 1 out]
                  }
                  frame #1 {
                    w506 = T8."Startup&Shutdown" ("Tab")
                    # "Turn off\nVelocity\non \nExit"
                    n192 = local write "ManualModeStop"(FALSE ("ManualModeStop")) -> ()
                    n193 = local write "Desired \nVelocity"(i16 0 ("Desired \nVelocity")) -> ()
                    n194 = local write "Local\nHeading"(i16 0 ("Local\nHeading")) -> ()
                    n195 = local write "Mode"(i16 0 ("Mode")) -> ()
                    n196 = local write "Tab"(w506) -> ()
                  }
                }
              }
            }
          }
          frame "AutoMode" {
            n197 = flat-sequence {
              tunnel: w514 -> [_]
              tunnel: [w517] -> w512
              tunnel: w511 -> [w517]
              tunnel: w510 -> [w516]
              tunnel: [w516] -> w509
              tunnel: w508 -> [_]
              tunnel: w512 -> [w524]
              tunnel: w509 -> [w522]
              tunnel: [w601] -> w515
              tunnel: [FALSE ("s")] -> w513
              frame #0 {
                # "Run Robot\nbased on\nmission\ndefinition\nfile"
                n198 = local write "AutoMissionMap"(w516) -> ()
                n199 = while {
                  shift-right: [w520] -> _
                  shift-left: _ -> [w519]
                  stop <- "RunAutoMode" continue-if-true
                  # "Wait for Run\nbutton press\nbefore\nturning on\nAutoMode\nCode"
                  n200 = Not(x=w519) -> (.not. x?=w520:bool)
                  n201 = Wait Until Next ms Multiple(millisecond multiple=u32 100 ("milliseconds to wait")) -> ()  [unwired: 1 out]
                  "Ready" <- w519
                }
              }
              frame #1 {
                n202 = while {
                  shift-right: [w570] -> _
                  shift-left: _ -> [w561]
                  tunnel: w524 -> [w565]
                  shift-right: [w563] -> _
                  shift-left: _ -> [w564]
                  tunnel: w522 -> [w556]
                  stop <- w560 stop-if-true
                  # "WhereAmI?"
                  n203 = local read "WhereAmI?FromBase"() -> (w555:T6)
                  n204 = Get Date/Time In Seconds "GetMiissionCurrentTime"() -> (seconds since 1Jan1904=w566:timestamp)
                  n205 = call "WhereForebrainPerception.vi"("Where? Midbrain"=w555) -> ("(xr,yr)"=w563:cluster{"X":dbl, "Y":dbl}, "Direction"=w549:dbl)  [unwired: 3 in, 2 out]
                  "Robot Position" <- w563
                  n206 = local read "RunAutoMode"() -> (w560:bool)
                  n207 = Greater Or Equal?(x=w549, y=181.0) -> (x >= y?=w553:bool)
                  n208 = To Double Precision Float(number=w566) -> (double precision float=w567:dbl)
                  n209 = Subtract(x=w567, y=w565) -> (x-y=w568:dbl)
                  n210 = Not(x=w561) -> (.not. x?=w570:bool)
                  n211 = call "DrawRobot.vi"("(xr,yr) old"=w564, "(xr,yr) new"=w563, "2D Picture"=w556) -> ("new picture"=→"AutoMissionMap":picture)
                  n212 = local read "SteerAngle"() -> (w558:dbl)
                  n213 = Divide(x=w568, y=60.0) -> (x/y=w562:dbl)
                  "MissionTimeAuto" <- w562
                  n214 = Subtract(x=w549, y=360.0) -> (x-y=w551:dbl)
                  n215 = Select(t=w551, s=w553, f=w549) -> (s? t:f=w550:dbl)
                  n216 = shared-variable "My Computer\\RobotBrainExLibrary.lvlib\\MissionTime"(w562) -> ()  [unwired: 1 in, 1 out]
                  n217 = Bundle("Direction"=w550, "SteerAngle"=w558) -> (→"A Heading":cluster{"Direction":dbl, "SteerAngle":dbl})  [unwired: 1 in]
                  n218 = Wait Until Next ms Multiple(millisecond multiple=u32 50 ("milliseconds to wait")) -> ()  [unwired: 1 out]
                  "Where?" <- w561
                }
                n219 = while {
                  shift-right: [w591] -> _
                  shift-left: _ -> [w590]
                  shift-right: [w573] -> _
                  shift-left: 0.0 ("SteerAngle") -> [w586]
                  stop <- w593 stop-if-true
                  # "needs to put out heading in local coordinates"
                  # "Think"
                  n220 = Not(x=w590) -> (.not. x?=w591:bool)
                  n221 = Or(x="Pause", y="E-Stop") -> (x .or. y?=w577:bool)
                  n222 = local read "WhereAmI?FromBase"() -> (w589:T6)
                  n223 = local read "WhatAroundMeMap?"() -> (w588:cluster{"T":dbl, "Range":dbl, "Bearing":dbl}[])
                  n224 = local read "MDF"() -> (w579:T4)
                  n225 = call "GotoWaypoint.vi"("InhibitIn"=w577, "CurrentSteerAngle"=w586, "WhatAroundMe? Clean"=w588, "WhereAmI? Clean"=w589, "MDF In"=w579) -> ("BehCom"=→"Current Behavior":T7, "MDF Out"=w581:T4, "ActCommand"=→"WayPointAct":dbl[], "Vel"=w574:dbl, "SteerAngle"=w573:dbl)  [unwired: 1 in, 1 out]
                  "SteerAngle" <- w573
                  "A Speed" <- w574
                  n226 = To Long Integer(number=w574) -> (32bit integer=w575:i32)
                  n227 = To Long Integer(number=w573) -> (32bit integer=w572:i32)
                  n228 = local write "MDF"(w581) -> ()
                  n229 = local write "Desired \nVelocity"(w575) -> ()
                  n230 = local read "RunAutoMode"() -> (w593:bool)
                  n231 = local write "Local\nHeading"(w572) -> ()
                  n232 = local read "MDF_Original"() -> (w584:T4)
                  n233 = local read "MDF"() -> (w583:T4)
                  n234 = Select(t=w584, s="Rerun MDF", f=w583) -> (s? t:f=w580:T4)
                  n235 = local write "MDF"(w580) -> ()
                  n236 = Wait Until Next ms Multiple(millisecond multiple=u32 50 ("milliseconds to wait")) -> ()  [unwired: 1 out]
                  "Neo-C" <- w590
                }
                n237 = while {
                  shift-right: [w542] -> _
                  shift-left: _ -> [w544]
                  stop <- w541 stop-if-true
                  # "WhatIsAroundMe?"
                  n238 = local read "WhatAroundMeMap?"() -> (w538:cluster{"T":dbl, "Range":dbl, "Bearing":dbl}[])
                  n239 = call "ProcessLidarData.vi"("WhatAroundMe?MM"=w538) -> ("Collision"=w539:bool, "data array [mag, phase (deg)]"=w543:cluster{"magnitude":dbl, "phase":dbl}[])
                  "CollisionLight 2" <- w539
                  n240 = local read "RunAutoMode"() -> (w541:bool)
                  n241 = call "SimLIDARPlot.vi"("data array [mag, phase (deg)]"=w543) -> ("SONAR"=→"AutoModeLIDAR":picture)  [unwired: 1 in]
                  n242 = Not(x=w544) -> (.not. x?=w542:bool)
                  "What?" <- w542
                  n243 = case shown="True" w539 {
                    frame False {
                      # "No \nBeep"
                    }
                    frame True {
                      n244 = call <vilib>:"Beep.vi"("use system alert? (T)"=TRUE, "duration (msec)"=u32 1000, "frequency (Hz)"=u32 900) -> ()  [unwired: 9 in]
                    }
                  }
                  n245 = Wait Until Next ms Multiple(millisecond multiple=u32 50 ("milliseconds to wait")) -> ()  [unwired: 1 out]
                }
                n246 = while {
                  shift-right: [w536] -> _
                  shift-left: _ -> [w535]
                  stop <- w534 stop-if-true
                  # "HowAmI?"
                  n247 = local read "Battery\nVolts"() -> (w532:i16)
                  n248 = local read "RunAutoMode"() -> (w534:bool)
                  n249 = Not(x=w535) -> (.not. x?=w536:bool)
                  n250 = Divide(x=w532, y=i16 1000) -> (x/y=→"AutoBattery":dbl)
                  n251 = Wait Until Next ms Multiple(millisecond multiple=u32 80 ("milliseconds to wait")) -> ()  [unwired: 1 out]
                  "How?" <- w535
                }
                n252 = while {
                  shift-right: [w529] -> _
                  shift-left: _ -> [w528]
                  stop <- w527 stop-if-true
                  # "calculate desired heading.vi"
                  # "see calc desired\nheading"
                  # "convert to \noutputtin\nDesired v and\nlocal heading"
                  # "chnage arbiter to be -180 to 180"
                  # "Note:\nadd other beh to\narbiter"
                  # "ForebrainAct"
                  n253 = local read "WayPointAct"() -> (w526:dbl[])
                  n254 = local read "RunAutoMode"() -> (w527:bool)
                  n255 = Not(x=w528) -> (.not. x?=w529:bool)
                  n256 = call "ForebrainArbiter.vi"("WaypointInput"=w526) -> ("ForebrainActCom"=w525:dbl[])  [unwired: 14 in]
                  n257 = shared-variable "My Computer\\RobotBrainExLibrary.lvlib\\ActCommand"(w525) -> ()  [unwired: 1 in, 1 out]
                  n258 = Wait Until Next ms Multiple(millisecond multiple=u32 50 ("milliseconds to wait")) -> ()  [unwired: 1 out]
                  "Act" <- w528
                }
              }
              frame #2 {
                w601 = T8."Startup&Shutdown" ("Tab")
                # "Set robot Vel to 0"
                # "Reset latched run\nswitch"
                # "Force control to\nShutdown Case"
                n259 = shared-variable "My Computer\\RobotBrainExLibrary.lvlib\\ForebrainCom"(T9 {"VelCom"=0.0, "BehCom"=enum."OpenFieldTransit"} ("ForebrainCom")) -> ()  [unwired: 1 in, 1 out]
                n260 = local write "RunAutoMode"(TRUE ("RunAutoMode")) -> ()
                n261 = Initialize Array(0.0 ("element"), 90 ("dimension size")) -> (w597:dbl[])
                n262 = shared-variable "My Computer\\RobotBrainExLibrary.lvlib\\ActCommand"(w597) -> ()  [unwired: 1 in, 1 out]
                n263 = shared-variable "My Computer\\RobotBrainExLibrary.lvlib\\Xstart"(200.0 ("Xstart")) -> ()  [unwired: 1 in, 1 out]
                n264 = shared-variable "My Computer\\RobotBrainExLibrary.lvlib\\Ystart"(400.0 ("Ystart")) -> ()  [unwired: 1 in, 1 out]
                n265 = local write "Tab"(w601) -> ()
              }
            }
          }
          frame "Documentation" {
            # "Add:\n1) Blinking lights in each loop to show that they are running"
            # "This mode is just a static data flow picture of the ForeBrain"
            n266 = Wait (ms)(milliseconds to wait=u32 500) -> ()  [unwired: 1 out]
          }
          frame "DebugTHINK" {
            w611 = T8."Startup&Shutdown" ("Tab")
            # "Add:\n1) a button for each midbrain behavior to help in debugging\n2) graph of \"neural\" arbiter brain waves for each actuator\n3) a button for each forebrain behavior"
            # "Put code here in place of delay"
            # "Sends Tab Control\nback to Startup\ncase"
            n267 = Wait (ms)(milliseconds to wait=u32 5000) -> ()  [unwired: 1 out]
            n268 = local write "Tab"(w611) -> ()
          }
          frame "Basic AutoMode" {
            # "Index of Destination Point"
            # "Where am I?\nDraw robots current location on map"
            n269 = local read "Tug X"() -> (w637:i32)
            n270 = local read "Tug Y"() -> (w638:i32)
            n271 = Bundle("Tug X"=w637, "Tug Y"=w638) -> (w636:cluster{"Tug X":i32, "Tug Y":i32})  [unwired: 1 in]
            n272 = call "DrawRobot.vi"("(xr,yr) old"=w636, "(xr,yr) new"=w636, "2D Picture"=w635) -> ("new picture"=→"BAM Mission Map":picture)
            n273 = local read "WhereAmI?FromBase"() -> (w641:T6)
            n274 = Unbundle(w641) -> ("X"=w618:dbl, "Y"=w617:dbl, "Direction"=w640:dbl)  [unwired: 1 out]
            "Pixel X" <- w618
            "Pixel Y" <- w617
            "Direction" <- w640
            n275 = call "rudderAngle.vi"("BoatHeading"=w640, "YGoal"="Pixel X Goal", "XGoal"="Pixel Y Goal", "Yboat"=w618, "Xboat"=w617) -> ("RudderAngle"=w626:i16)  [unwired: 1 in, 2 out]
            n276 = call "NearWaypointTest.vi"("Yrobot"=w617, "Xrobot"=w618, "Ywaypoint"="Pixel Y Goal", "Xwaypoiny"="Pixel X Goal") -> ("AtWaypoint"=w614:bool)  [unwired: 7 in]
            n277 = Select(t="Heading", s="Manual Override", f=w626) -> (s? t:f=w625:i16)
            n278 = Select(t="Velocity", s="Manual Override", f=i16 8 ("t")) -> (s? t:f=w616:i16)
            n279 = local read "Battery\nVolts"() -> (w633:i16)
            n280 = Select(t=i16 7, s=w614, f=w616) -> (s? t:f=w613:i16)
            n281 = local write "Local\nHeading"(w625) -> ()
            n282 = local write "Desired \nVelocity"(w613) -> ()
            n283 = Divide(x=w633, y=1000) -> (x/y=→"Battery Level":dbl)
            n284 = local read "Tab"() -> (w629:T1)
          }
        }
        n285 = Not(x=w194) -> (.not. x?=w178:bool)
        "Robot Live" <- w178
      }
      n286 = while {
        tunnel: w57 -> [w160]
        tunnel: w56 -> [w159]
        tunnel: [w158] -> w54
        tunnel: [w157] -> w55
        shift-right: [w151] -> _
        shift-left: _ -> [w150]
        stop <- w161 continue-if-true
        w163 = 250  # timeout
        # "Finds and displays tugs position"
        # "runs continuously till program stops"
        # "Comminications with Base Station"
        # "receive string"
        # "If time out, post timeout and\nremove the timeout error"
        # "Read data from the port."
        n287 = Wait Until Next ms Multiple(millisecond multiple=u32 1) -> ()  [unwired: 1 out]
        n288 = UDP Read(connection ID=w160, timeout ms (25000)=w163, 8:w159) -> (data out=w152:string, error out=w164:errorcluster, 3:w157:refnum<k16>)  [unwired: 1 in, 2 out]
        "Base Station String" <- w152
        n289 = local write "Base Station data rec'd"(w152) -> ()
        n290 = Unbundle By Name(w164) -> ("code"=w167:i32)
        n291 = Equal?(x=w167, y=56) -> (x = y?=w165:bool)
        "BS Time Out?" <- w165
        n292 = case shown="True" w165 {
          tunnel: [w174 errorcluster {"status"=FALSE, "code"=0, "source"=""} ("error out")] -> w158
          tunnel: w164 -> [w174 _]
          frame False {
          }
          frame True {
          }
        }
        n293 = call "PC parse the data.vi"("Nav String"=w152, "Tug"="Tug letter") -> ("Buoy locations"=w156:cluster{"regular expression":string, i32, i32}[], "Tug Location"=w154:T14, "Valid?"=w155:bool)  [unwired: 1 out]
        "Valid ?" <- w155
        n294 = local write "Buoy locations"(w156) -> ()
        n295 = case shown="True" w155 {
          tunnel: w154 -> [_ w173]
          frame False {
            # "No \nchange"
          }
          frame True {
            # "New values from BaseStation"
            n296 = shared-variable "My Computer\\RobotBrainExLibrary.lvlib\\MissionTime"() -> (w172:dbl)  [unwired: 1 in, 1 out]
            n297 = Unbundle(w173) -> (w171:i32, w170:i32, w169:i32)  [unwired: 1 out]
            n298 = local write "Tug X"(w171) -> ()
            n299 = local write "Tug Y"(w170) -> ()
            n300 = local write "Tug H"(w169) -> ()
            n301 = Bundle(w172, w171, w170, w169) -> (w168:cluster{dbl, i32, i32, i32})  [unwired: 1 in]
            n302 = local write "WhereAmI?FromBase"(w168) -> ()
          }
        }
        n303 = local read "RunRobot"() -> (w161:bool)
        n304 = Not(x=w150) -> (.not. x?=w151:bool)
        "udp rate" <- w150
      }
      n305 = while {
        tunnel: w58 -> [_]
        stop <- w100 continue-if-true
        n306 = local read "Upper Midbrain Active"() -> (w99:bool)
        n307 = case shown="True" w99 {
          frame False {
            # "loop timimng \ncontrolled externally"
            # "Send commands to NXT"
            n308 = local read "Desired \nVelocity"() -> (w111:i16)
            n309 = local read "Local\nHeading"() -> (w110:i16)
            n310 = local read "Mode"() -> (w109:i16)
            n311 = case shown="2" w109 {
              tunnel: w111 -> [w114 w125 w132]
              tunnel: w110 -> [w113 w124 w133]
              tunnel: [w115 w120 w128] -> w103
              tunnel: i16 7 ("element") -> [w112 w121 w129]
              frame 0, Default {
                w116 = i16 0 ("element")
                n312 = Build Array(u8 91 ("element"), w112, w113, w114, i16 1 ("element"), w116, w116, w116, w116, w116, u8 93 ("element")) -> (w115:i16[])
              }
              frame 1 {
                w122 = i16 0 ("element")
                n313 = Build Array(u8 91 ("element"), w121, w124, w125, w122, i16 1 ("element"), w122, w122, w122, w122, u8 93 ("element")) -> (w120:i16[])
              }
              frame 2 {
                w130 = i16 0 ("element")
                n314 = Build Array(u8 91 ("element"), w129, w133, w132, w130, w130, i16 1 ("element"), w130, w130, w130, u8 93 ("element")) -> (w128:i16[])
              }
            }
            n315 = Select(t=u8[] [91, 7, 7, 7, 1, 0, 0, 0, 0, 0, 92], s="Soft E-Stop", f=w103) -> (s? t:f=w104:i16[])
            n316 = Add(x=w104, y=u8[] [0, 65, 65, 65, 65, 65, 65, 65, 65, 65, 0]) -> (x+y=w105:i16[])
            n317 = Byte Array To String(unsigned byte array=w105) -> (string=w102:string)
            n318 = local write "Send String"(w102) -> ()
          }
          frame True {
            n319 = local read "ManualModeStop"() -> (w137:bool)
            n320 = call "UpperMidbrain.vi"("SOFT E-STOP"=w137, "IR Servo"=u8 7) -> ("string"=w138:string)  [unwired: 9 in]
            n321 = local write "Send String"(w138) -> ()
          }
        }
        n322 = local read "RunRobot"() -> (w100:bool)
      }
      n323 = while {
        tunnel: w58 -> [_]
        stop <- w77 continue-if-true
        # "Receive information from NXT"
        n324 = local read "String Received"() -> (w82:string)
        n325 = Wait Until Next ms Multiple(millisecond multiple=u32 100) -> ()  [unwired: 1 out]
        n326 = String Subset(string=w82, offset (0)=1, length (rest)=1 ("length (rest)")) -> (substring=w81:string)
        n327 = case shown="\"N\"" w81 {
          tunnel: w82 -> [_ w84]
          frame Default {
          }
          frame "N" {
            # "0-15"
            # "Parse command \"N\""
            n328 = String Subset(string=w84, offset (0)=2, length (rest)=4 ("length (rest)")) -> (substring=w95:string)
            n329 = String Subset(string=w84, offset (0)=6, length (rest)=3 ("length (rest)")) -> (substring=w91:string)
            n330 = String Subset(string=w84, offset (0)=9, length (rest)=2 ("length (rest)")) -> (substring=w87:string)
            n331 = Decimal String To Number(string=w95) -> (number=w98:i32)  [unwired: 2 in, 1 out]
            n332 = Decimal String To Number(string=w91) -> (number=w90:i32)  [unwired: 2 in, 1 out]
            n333 = Decimal String To Number(string=w87) -> (number=w88:i32)  [unwired: 2 in, 1 out]
            n334 = To Word Integer(number=w98) -> (16bit integer=w94:i16)
            n335 = To Word Integer(number=w90) -> (16bit integer=w89:i16)
            n336 = To Long Integer(number=w88) -> (32bit integer=w83:i32)
            n337 = local write "LidarDist"(w89) -> ()
            n338 = local write "Battery\nVolts"(w94) -> ()
            n339 = local write "IR Index"(w83) -> ()
          }
        }
        n340 = local read "RunRobot"() -> (w77:bool)
      }
      n341 = while {
        stop <- w76 continue-if-true
        # "Run Simulated MapDAR"
        n342 = local read "Tug X"() -> (w74:i32)
        n343 = local read "Tug Y"() -> (w73:i32)
        n344 = local read "Tug H"() -> (w72:i32)
        n345 = Bundle "Bundle"("Tug X"=w74, "Tug Y"=w73, "Tug H"=w72) -> (w75:cluster{"Tug X":i32, "Tug Y":i32, "Tug H":i32})  [unwired: 1 in]
        n346 = call "HindbrainLIDAR_Sim.vi"("SubPosition"=w75) -> ("WhatAroundMe?"=→"WhatAroundMeMap?":cluster{"T":dbl, "Range":dbl, "Bearing":dbl}[])  [unwired: 10 in]
        n347 = local read "RunRobot"() -> (w76:bool)
      }
    }
    frame #2 {
      # "Close XBee Radio"
      # "Close UDP port"
      # "Realease LIDAR\nMemory"
      # "Reset Run \nSwitch"
      # "Shutdown Robot"
      n348 = call "Pixel_LIDAR_Close.vi"("error in (no error) 2"=w646, "Image"=w647) -> ()  [unwired: 1 in]
      n349 = local write "RunRobot"(TRUE ("RunRobot")) -> ()
      n350 = call "XB PC Close.vi"("error in (no error)"=w644, "VISA resource name"=w645) -> ()
      n351 = UDP Close(connection ID=w643, 8:w642) -> ()  [unwired: 2 out]
      "error out" <- w644
    }
  }
